vi "Init6363IO.vi"(8 "error in":errorcluster caption="错误输入") -> (0 "error out":errorcluster caption="错误输出", 3 "task out":refnum<k21> caption="任务输出")   [LabVIEW 2014]
uses:
  <vilib>/DAQmx/create/channels.llb/DAQmx Create Channel (DO-Digital Output).vi
  <resource>/objmgr/daqmx.rc
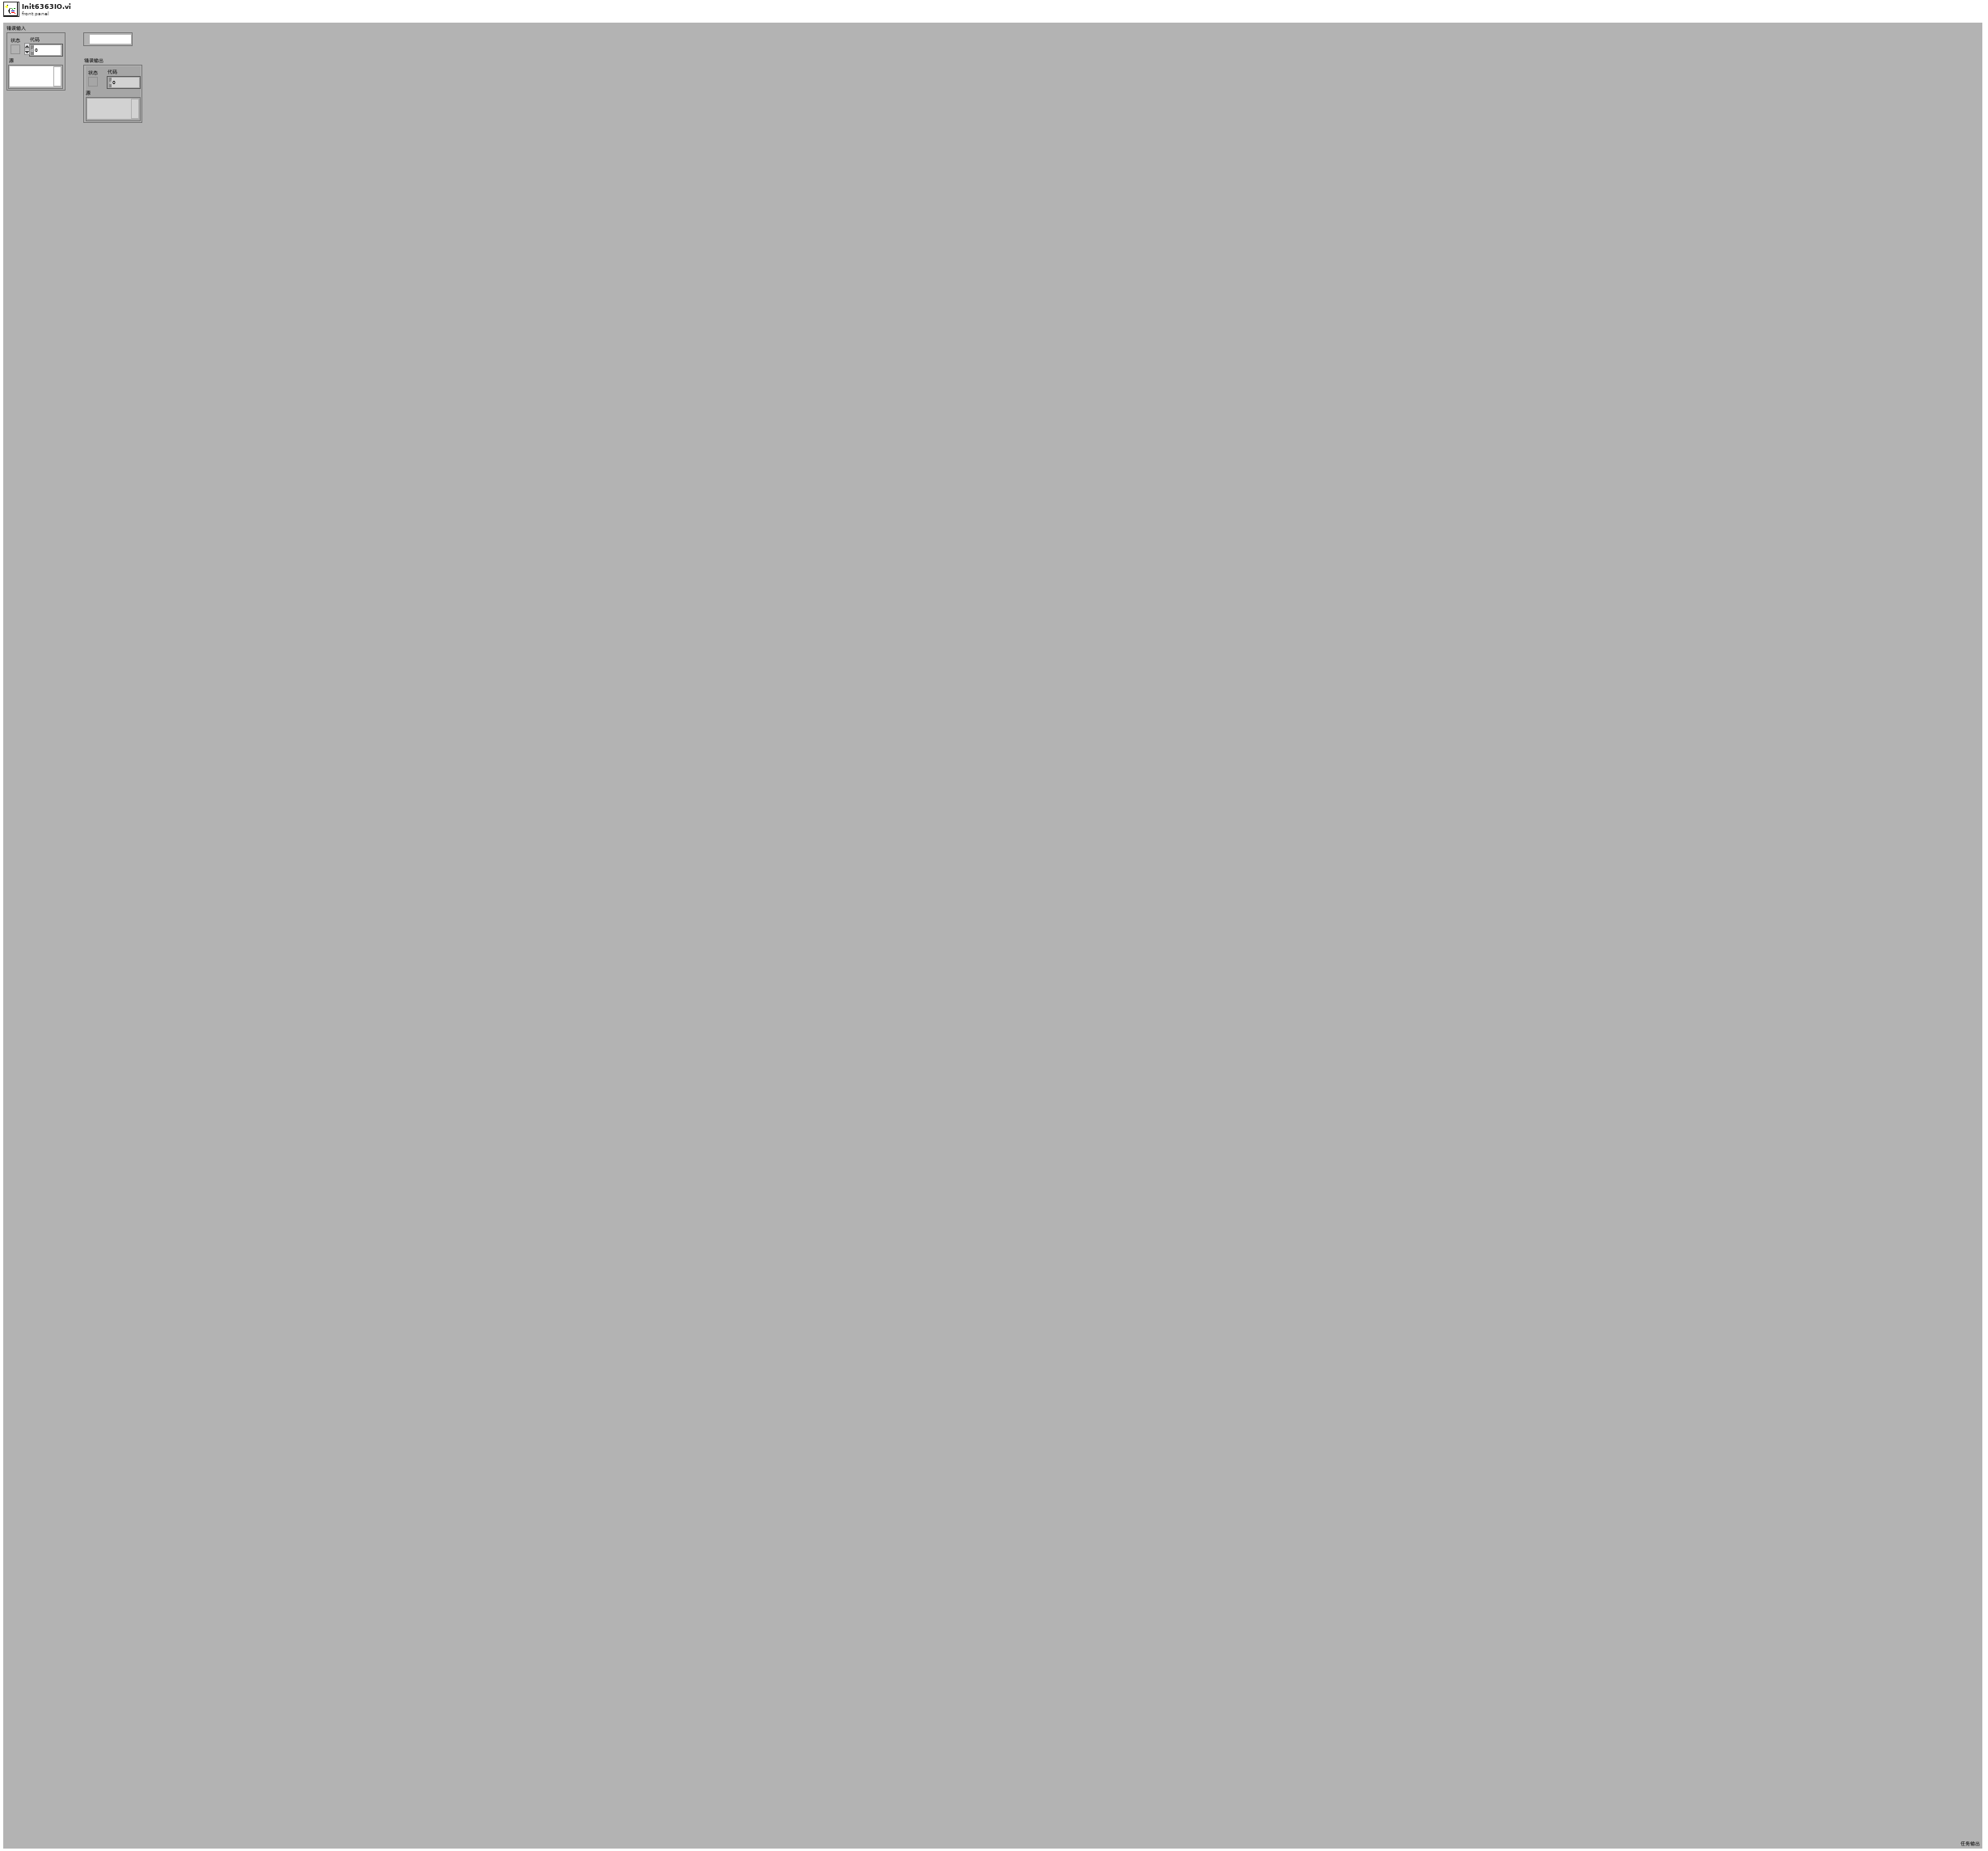
[diagram p1: front panel]
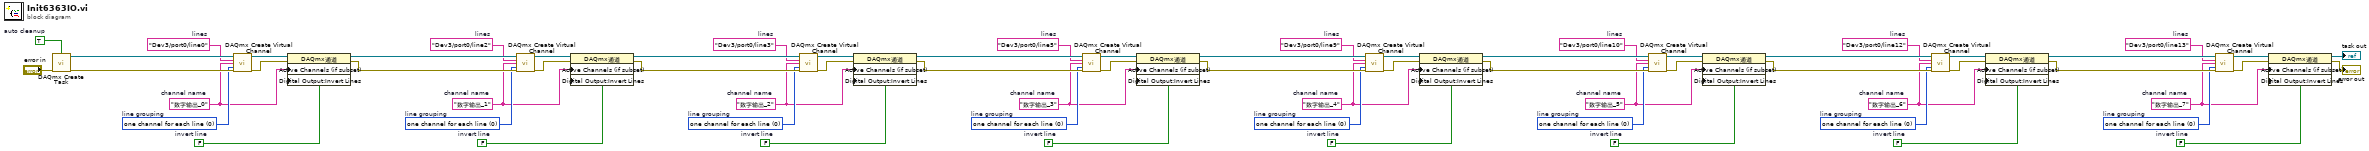
[diagram p0: block diagram]
diagram:
  w2 = FALSE  # invert line
  w7 = 0 items=["one channel for each line", "one channel for all lines"]  # line grouping
  w1 = "数字输出_7"  # channel name
  w8 = "Dev3/port0/line13"  # lines
  w11 = FALSE  # invert line
  w15 = 0 items=["one channel for each line", "one channel for all lines"]  # line grouping
  w10 = "数字输出_6"  # channel name
  w16 = "Dev3/port0/line12"  # lines
  w19 = FALSE  # invert line
  w23 = 0 items=["one channel for each line", "one channel for all lines"]  # line grouping
  w18 = "数字输出_5"  # channel name
  w24 = "Dev3/port0/line10"  # lines
  w27 = FALSE  # invert line
  w31 = 0 items=["one channel for each line", "one channel for all lines"]  # line grouping
  w26 = "数字输出_4"  # channel name
  w32 = "Dev3/port0/line9"  # lines
  w35 = FALSE  # invert line
  w39 = 0 items=["one channel for each line", "one channel for all lines"]  # line grouping
  w34 = "数字输出_3"  # channel name
  w40 = "Dev3/port0/line5"  # lines
  w43 = FALSE  # invert line
  w47 = 0 items=["one channel for each line", "one channel for all lines"]  # line grouping
  w42 = "数字输出_2"  # channel name
  w48 = "Dev3/port0/line3"  # lines
  w51 = FALSE  # invert line
  w55 = 0 items=["one channel for each line", "one channel for all lines"]  # line grouping
  w50 = "数字输出_1"  # channel name
  w56 = "Dev3/port0/line2"  # lines
  w59 = FALSE  # invert line
  w63 = 0 items=["one channel for each line", "one channel for all lines"]  # line grouping
  w58 = "数字输出_0"  # channel name
  w64 = "Dev3/port0/line0"  # lines
  w66 = TRUE  # auto cleanup
  n1 = call <vilib>:"DAQmx Create Task.vi"("auto cleanup"=w66, "error in"="error in") -> ("task out"=w65:refnum<k21>, "error out"=w67:errorcluster)  [unwired: 12 in]
  n2 = call-poly <vilib>:"DAQmx Create Virtual Channel.vi"("task in"=w65, "lines"=w64, "name to assign"=w58, "line grouping"=w63, "error in"=w67) -> ("task out"=w62:refnum<k21>, "error out"=w61:errorcluster)  [unwired: 9 in]
  n3 = property class="DAQmx通道"(reference=w62, error in=w61, "Active Channels (if subset)"=w58, "Digital Output:Invert Lines"=w59) -> (reference out=w57:refnum<k21>, error out=w60:errorcluster)
  n4 = call-poly <vilib>:"DAQmx Create Virtual Channel.vi"("task in"=w57, "lines"=w56, "name to assign"=w50, "line grouping"=w55, "error in"=w60) -> ("task out"=w54:refnum<k21>, "error out"=w53:errorcluster)  [unwired: 9 in]
  n5 = property class="DAQmx通道"(reference=w54, error in=w53, "Active Channels (if subset)"=w50, "Digital Output:Invert Lines"=w51) -> (reference out=w49:refnum<k21>, error out=w52:errorcluster)
  n6 = call-poly <vilib>:"DAQmx Create Virtual Channel.vi"("task in"=w49, "lines"=w48, "name to assign"=w42, "line grouping"=w47, "error in"=w52) -> ("task out"=w46:refnum<k21>, "error out"=w45:errorcluster)  [unwired: 9 in]
  n7 = property class="DAQmx通道"(reference=w46, error in=w45, "Active Channels (if subset)"=w42, "Digital Output:Invert Lines"=w43) -> (reference out=w41:refnum<k21>, error out=w44:errorcluster)
  n8 = call-poly <vilib>:"DAQmx Create Virtual Channel.vi"("task in"=w41, "lines"=w40, "name to assign"=w34, "line grouping"=w39, "error in"=w44) -> ("task out"=w38:refnum<k21>, "error out"=w37:errorcluster)  [unwired: 9 in]
  n9 = property class="DAQmx通道"(reference=w38, error in=w37, "Active Channels (if subset)"=w34, "Digital Output:Invert Lines"=w35) -> (reference out=w33:refnum<k21>, error out=w36:errorcluster)
  n10 = call-poly <vilib>:"DAQmx Create Virtual Channel.vi"("task in"=w33, "lines"=w32, "name to assign"=w26, "line grouping"=w31, "error in"=w36) -> ("task out"=w30:refnum<k21>, "error out"=w29:errorcluster)  [unwired: 9 in]
  n11 = property class="DAQmx通道"(reference=w30, error in=w29, "Active Channels (if subset)"=w26, "Digital Output:Invert Lines"=w27) -> (reference out=w25:refnum<k21>, error out=w28:errorcluster)
  n12 = call-poly <vilib>:"DAQmx Create Virtual Channel.vi"("task in"=w25, "lines"=w24, "name to assign"=w18, "line grouping"=w23, "error in"=w28) -> ("task out"=w22:refnum<k21>, "error out"=w21:errorcluster)  [unwired: 9 in]
  n13 = property class="DAQmx通道"(reference=w22, error in=w21, "Active Channels (if subset)"=w18, "Digital Output:Invert Lines"=w19) -> (reference out=w17:refnum<k21>, error out=w20:errorcluster)
  n14 = call-poly <vilib>:"DAQmx Create Virtual Channel.vi"("task in"=w17, "lines"=w16, "name to assign"=w10, "line grouping"=w15, "error in"=w20) -> ("task out"=w14:refnum<k21>, "error out"=w13:errorcluster)  [unwired: 9 in]
  n15 = property class="DAQmx通道"(reference=w14, error in=w13, "Active Channels (if subset)"=w10, "Digital Output:Invert Lines"=w11) -> (reference out=w9:refnum<k21>, error out=w12:errorcluster)
  n16 = call-poly <vilib>:"DAQmx Create Virtual Channel.vi"("task in"=w9, "lines"=w8, "name to assign"=w1, "line grouping"=w7, "error in"=w12) -> ("task out"=w6:refnum<k21>, "error out"=w5:errorcluster)  [unwired: 9 in]
  n17 = property class="DAQmx通道"(reference=w6, error in=w5, "Active Channels (if subset)"=w1, "Digital Output:Invert Lines"=w2) -> (reference out=→"task out":refnum<k21>, error out=→"error out":errorcluster)
